vi "Invoke-error.vi"(6 "Error":T1, 8 "error in (no error)":errorcluster, 9 "Overwrite?":bool, 10 "Additional message":string) -> (0 "error out":errorcluster)   [LabVIEW 2013, in "SLMServer.lvlib" / "SLMServer.lvclass"]
uses:
  SLMServer.lvclass
  Custom-errors.ctl
  <vilib>/Utility/error.llb/DialogType.ctl
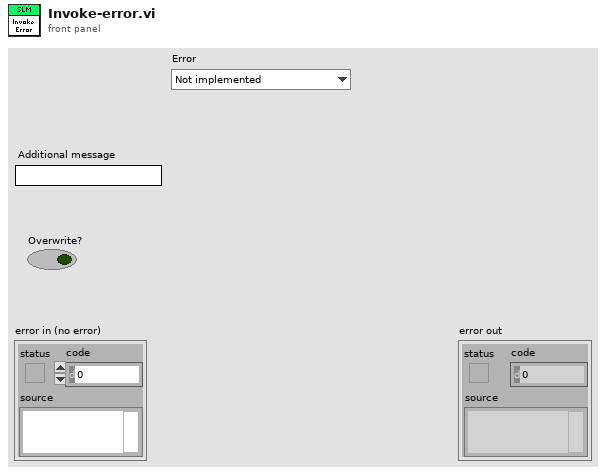
[diagram p1: front panel]
types:
  T1 = typedef "SLMServer.lvlib/SLMServer.lvclass/Custom-errors.ctl" = enum16{"Not implemented", "Command not recognized", "Invalid input", "Timeout", "Client not allowed", "Max clients reached"}
  T2 = typedef "DialogType.ctl" = u16
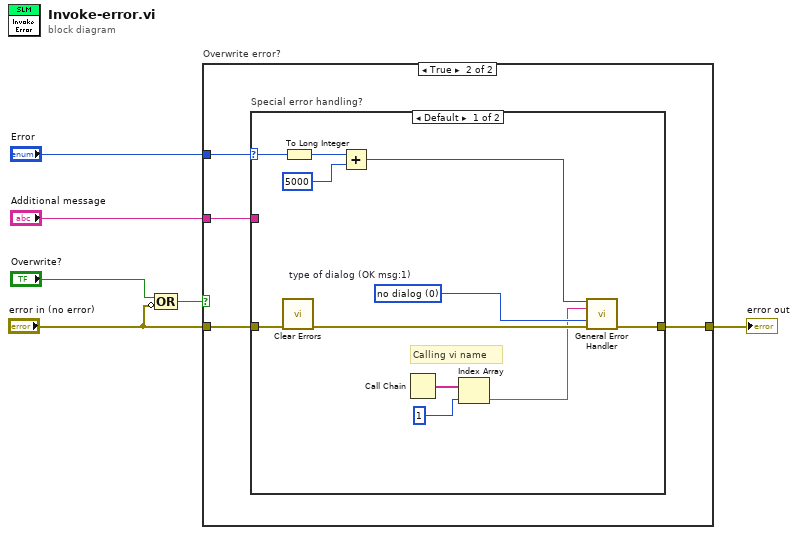
[diagram p0: block diagram]
diagram:
  n1 = Compound Arithmetic op=OR("Overwrite?", invert "error in (no error)") -> (w2:bool)
  n2 = case "Overwrite error?" shown="True" w2 {
    tunnel: [w7 w8] -> w6
    tunnel: "Error" -> [_ w11]
    tunnel: "Additional message" -> [_ w10]
    tunnel: "error in (no error)" -> [w7 w9]
    frame False {
    }
    frame True {
      n3 = case "Special error handling?" shown="Default" w11 {
        selector: w11 -> [w19 _]
        tunnel: [w22 w23] -> w8
        tunnel: w10 -> [_ _]
        tunnel: w9 -> [w16 w23]
        frame Default {
          w18 = T2 0 items=["no dialog", "OK message", "continue or stop message", "OK message + warnings", "continue/stop + warnings"]  # type of dialog (OK msg:1)
          # "Calling vi name"
          n4 = call <vilib>:"Clear Errors.vi"("error in (no error)"=w16) -> ("error out"=w15:errorcluster)  [unwired: 6 in]
          n5 = To Long Integer(number=w19) -> (32bit integer=w17:i32)
          n6 = Add(x=w17, y=5000) -> (x+y=w21:i32)
          n7 = Call Chain() -> (call chain=w14:string[])
          n8 = Index Array(array=w14, index=1) -> (element=w12:string)
          n9 = call <vilib>:"General Error Handler.vi"("[error code] (0)"=w21, "[error source] (\" \")"=w12, "type of dialog (OK msg:1)"=w18, "error in (no error)"=w15) -> ("error out"=w22:errorcluster)  [unwired: 7 in, 4 out]
        }
        frame "Not implemented" {
          # "No error."
        }
      }
    }
  }
  "error out" <- w6
